vi "construct.vi"(8 "error in (no error)":errorcluster, 9 "price":dbl, 10 "id":u32) -> (0 "error out":errorcluster, 3 "Chair out":refnum<class "Chair.lvclass">)   [LabVIEW 2021, in "Chair.lvclass"]
uses:
  Chair.lvclass
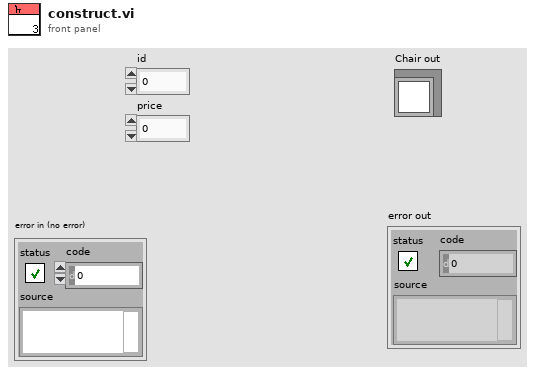
[diagram p1: front panel]
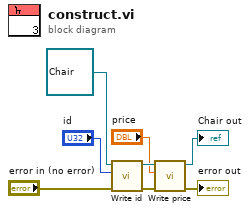
[diagram p0: block diagram]
diagram:
  n1 = call-dynamic "Write id.vi"("error in (no error)"="error in (no error)", "id"="id", "Furniture in"=refnum<class "Chair.lvclass"> refnum ("Chair.lvclass")) -> ("error out"=w3:errorcluster, "Furniture out"=w7:refnum<class "Chair.lvclass">)  [unwired: 7 in]
  n2 = call-dynamic "Write price.vi"("error in (no error)"=w3, "price"="price", "Furniture in"=w7) -> ("error out"=→"error out":errorcluster, "Furniture out"=→"Chair out":refnum<class "Chair.lvclass">)  [unwired: 7 in]
